vi "Filename.vi"(6 "Densities and De Boer":cluster{"Array":dbl[], "Array":dbl[]}[](array[cluster]), 8 "error in (no error)":errorcluster, 9 "P Graph and Intensities and RF":cluster{"Array":dbl[], "Array":dbl[]}[](array[cluster]), 10 "Q Graph":cluster{"Array":dbl[], "Array 2":dbl[]}, 11 "Byte Stream File in":refnum<file>) -> (0 "error out":errorcluster, 3 "Byte Stream File out":refnum<file>)   [LabVIEW 2018]
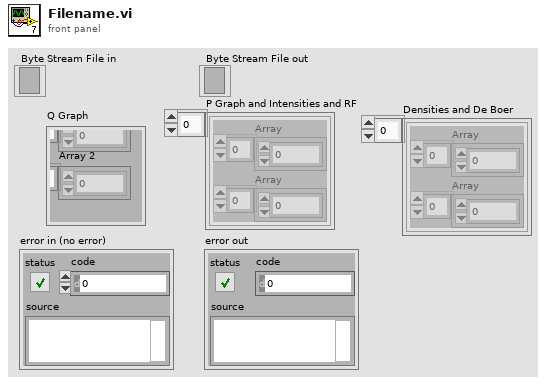
[diagram p1: front panel]
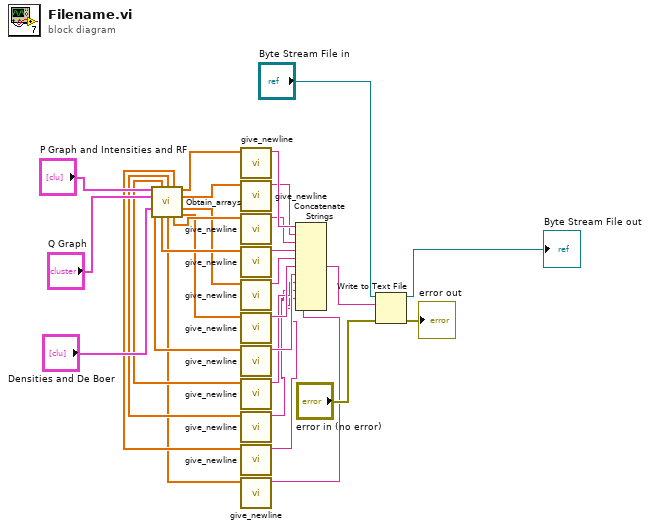
[diagram p0: block diagram]
diagram:
  n1 = call "Obtain_arrays.vi"("P Graph and Intensities and RF"="P Graph and Intensities and RF", "Q Graph"="Q Graph", "Densities and De Boer"="Densities and De Boer") -> ("rho+"=w8:dbl[], "rho0"=w7:dbl[], "rho-"=w6:dbl[], "P"=w16:dbl[], "Q"=w15:dbl[], "RF Range 1"=w12:dbl[], "AFP Range"=w10:dbl[], "I-"=w13:dbl[], "De Boer"=w5:dbl[], "I+"=w14:dbl[], "RF Range 2"=w11:dbl[])  [unwired: 2 in]
  n2 = call "give_newline.vi"("Array for writing"=w16) -> ("To file with newline"=w23:string)  [unwired: 10 in]
  n3 = call "give_newline.vi"("Array for writing"=w15) -> ("To file with newline"=w22:string)  [unwired: 10 in]
  n4 = call "give_newline.vi"("Array for writing"=w14) -> ("To file with newline"=w21:string)  [unwired: 10 in]
  n5 = call "give_newline.vi"("Array for writing"=w13) -> ("To file with newline"=w20:string)  [unwired: 10 in]
  n6 = call "give_newline.vi"("Array for writing"=w12) -> ("To file with newline"=w19:string)  [unwired: 10 in]
  n7 = call "give_newline.vi"("Array for writing"=w11) -> ("To file with newline"=w18:string)  [unwired: 10 in]
  n8 = call "give_newline.vi"("Array for writing"=w10) -> ("To file with newline"=w17:string)  [unwired: 10 in]
  n9 = call "give_newline.vi"("Array for writing"=w8) -> ("To file with newline"=w4:string)  [unwired: 10 in]
  n10 = call "give_newline.vi"("Array for writing"=w7) -> ("To file with newline"=w3:string)  [unwired: 10 in]
  n11 = call "give_newline.vi"("Array for writing"=w6) -> ("To file with newline"=w2:string)  [unwired: 10 in]
  n12 = call "give_newline.vi"("Array for writing"=w5) -> ("To file with newline"=w1:string)  [unwired: 10 in]
  n13 = Concatenate Strings(w23, w22, w21, w20, w19, w18, w17, w4, w3, w2, w1) -> (w24:string)
  n14 = Write to Text File(file (use dialog)="Byte Stream File in", text=w24, error in="error in (no error)") -> (refnum out=→"Byte Stream File out":refnum<file>, error out=→"error out":errorcluster)  [unwired: 1 in, 1 out]
